vi "2.A-Spoof Reality.vi"() -> ()   [LabVIEW 2011]
uses:
  2 Typedefs/2.A.1-Spoof Reality State.ctl
  2 Globals/2 Global.vi
panel:
  out "Velocity internal":dbl[](array[numeric])
  out "Perceived Wind":cluster{"X Position":dbl, "Y Position":dbl}
  out "Position":cluster{"X Position":dbl, "Y Position":dbl}
  out "Global Wind":cluster{"X Position":dbl, "Y Position":dbl}
  in  "Wind Angle":dbl
  out "Orientation":cluster{"X Position":dbl, "Y Position":dbl}
  in  "Stop Spoofing Reality":bool
  out "XY Graph":cluster{dbl, dbl}[](graph)
  out "Speed:":dbl
  in  "Wind Speed":dbl
  # "This is the Bass. It's catchy. You like it."
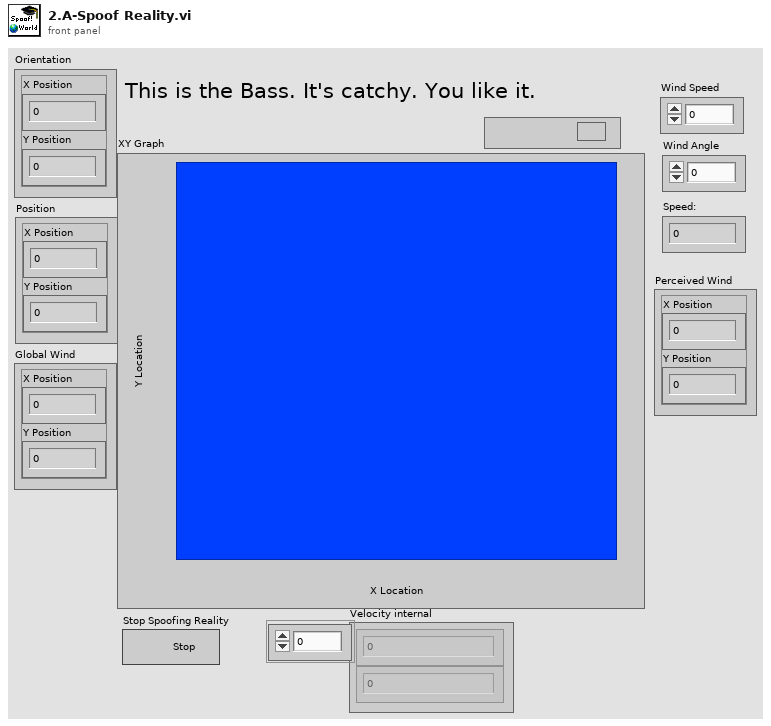
[diagram p1: front panel]
types:
  T1 = typedef "2.A.1-Spoof Reality State.ctl" = enum16{"Spoof Reality", "Think"}
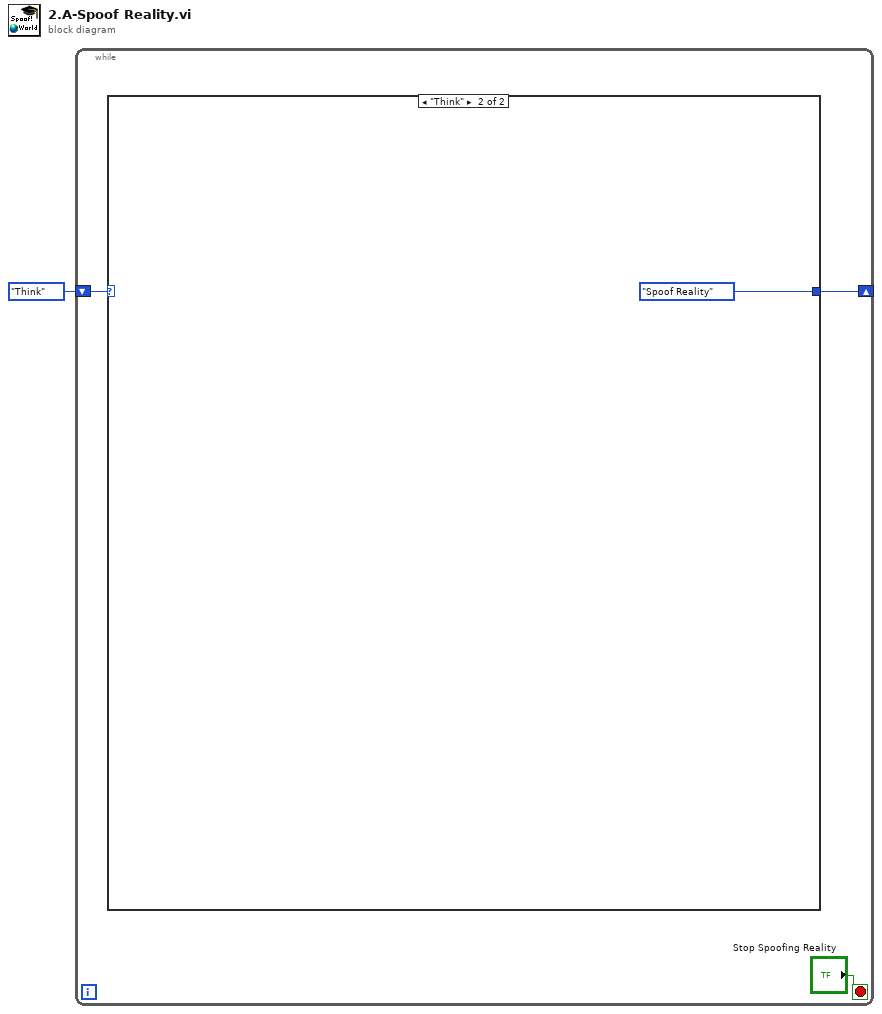
[diagram p0: block diagram]
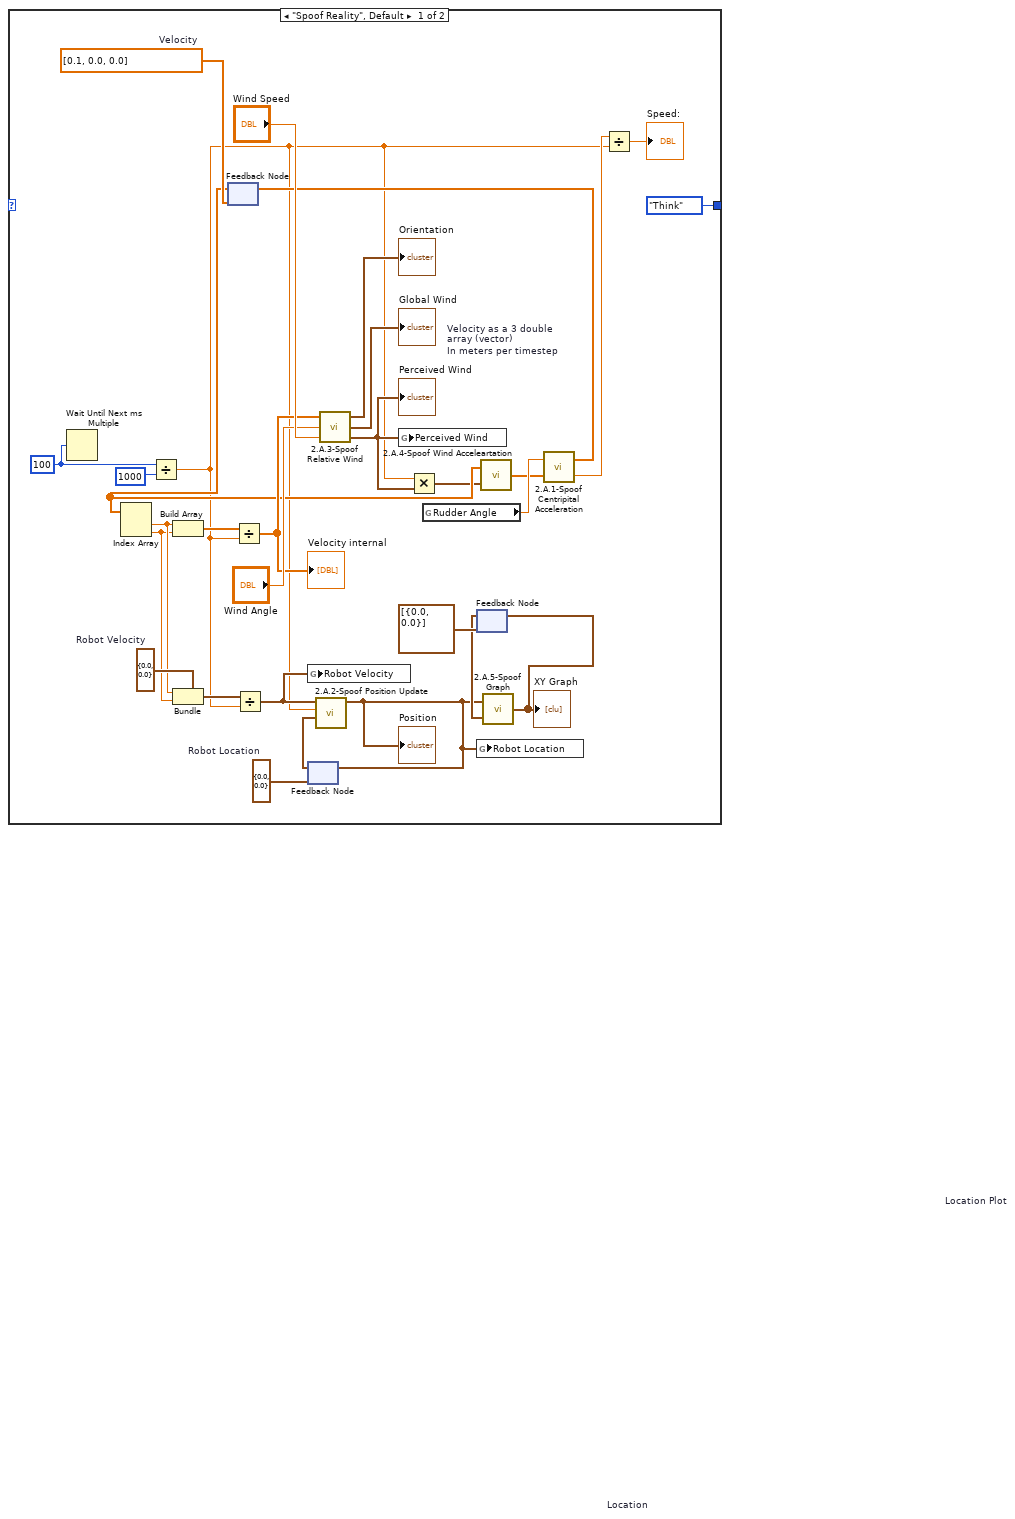
[diagram p2: hidden frame]
diagram:
  n1 = while {
    shift-right: [w2] -> _
    shift-left: 2.A.1-Spoof_Reality_State."Think" -> [w3]
    stop <- "Stop Spoofing Reality" stop-if-true
    n2 = case shown="\"Think\"" w3 {
      tunnel: [2.A.1-Spoof_Reality_State."Think" 2.A.1-Spoof_Reality_State."Spoof Reality"] -> w2
      frame "Spoof Reality", Default {
        w18 = dbl[] [0.1, 0.0, 0.0]  # Velocity
        w19 = cluster{"X Position":dbl, "Y Position":dbl} {"X Position"=0.0, "Y Position"=0.0}  # Robot Velocity
        w29 = cluster{"X Position":dbl, "Y Position":dbl} {"X Position"=0.0, "Y Position"=0.0}  # Robot Location
        w21 = u32 100 ("millisecond multiple")
        n3 = Wait Until Next ms Multiple(millisecond multiple=w21) -> ()  [unwired: 1 out]
        n4 = Divide(x=w21, y=u32 1000 ("x")) -> (x/y=w5:dbl)
        n5 = feedback #1 "Velocity as a 3 double array (vector)\nIn meters per timestep"(w18) -> (w10:dbl[])
        n6 = Index Array(array=w10) -> (element #1=w15:dbl, element #2=w14:dbl)  [unwired: 2 in]
        n7 = Build Array(w15, w14) -> (w13:dbl[])
        n8 = Bundle(cluster=w19, "X Position"=w15, "Y Position"=w14) -> (w17:cluster{"X Position":dbl, "Y Position":dbl})
        n9 = Divide(x=w13, y=w5) -> (x/y=w12:dbl[])
        "Velocity internal" <- w12
        n10 = Divide(x=w17, y=w5) -> (x/y=w11:cluster{"X Position":dbl, "Y Position":dbl})
        n11 = global write "2 Global.vi" "Robot Velocity"(w11) -> ()
        n12 = feedback #2 "Location"(w29) -> (w28:cluster{"X Position":dbl, "Y Position":dbl})
        n13 = call "2.A.2-Spoof Position Update.vi"("Old Position"=w28, "dt"=w5, "Robot Velocity"=w11) -> ("New Position"=w24:cluster{"X Position":dbl, "Y Position":dbl})  [unwired: 8 in]
        "Position" <- w24
        n14 = feedback-in #2(w24) -> ()
        n15 = call "2.A.3-Spoof Relative Wind.vi"("Wind Speed"="Wind Speed", "Wind Angle"="Wind Angle", "Velocity (3 array)"=w12) -> ("Perceived Wind"=w8:cluster{"X Position":dbl, "Y Position":dbl}, "Global Wind"=→"Global Wind":cluster{"X Position":dbl, "Y Position":dbl}, "Orientation"=→"Orientation":cluster{"X Position":dbl, "Y Position":dbl})
        "Perceived Wind" <- w8
        n16 = global write "2 Global.vi" "Perceived Wind"(w8) -> ()
        n17 = Multiply(x=w5, y=w8) -> (x*y=w7:cluster{"X Position":dbl, "Y Position":dbl})
        n18 = global read "2 Global.vi" "Rudder Angle"() -> (w23:dbl)
        n19 = feedback #3 "Location Plot"(cluster{dbl, dbl}[] [{0.0, 0.0}] ("XY Graph")) -> (w25:cluster{dbl, dbl}[])
        n20 = global write "2 Global.vi" "Robot Location"(w24) -> ()
        n21 = call "2.A.4-Spoof Wind Acceleartation.vi"("Perceived Wind"=w7, "Old Velocity"=w10) -> ("New Velocity"=w9:dbl[])
        n22 = call "2.A.5-Spoof Graph.vi"("XY Graph"=w25, "New Position"=w24) -> ("Array"=w26:cluster{"X Position":dbl, "Y Position":dbl}[])
        "XY Graph" <- w26
        n23 = feedback-in #3(w26) -> ()
        n24 = call "2.A.1-Spoof Centripital Acceleration.vi"("Old Velocity"=w9, "Rudder Angle"=w23) -> ("Speed"=w16:dbl, "New Velocity"=w22:dbl[])
        n25 = feedback-in #1(w22) -> ()
        n26 = Divide(x=w16, y=w5) -> (x/y=→"Speed:":dbl)
      }
      frame "Think" {
      }
    }
  }
